vi "fi-constructor.vi"(7 "table.ref in":refnum<vi>, 8 "error in (no error)":errorcluster, 11 "frameInput in":refnum<class "bFrameIO.lvclass">) -> (0 "error out":errorcluster, 3 "frameInput out":refnum<class "bFrameIO.lvclass">)   [LabVIEW 2015, in "bFrameIO.lvclass"]
uses:
  bFrameIO.lvclass
  class.can.table/CAN_table.ctl
  controls/input.params.ctl
  controls/input-states.ctl
  <vilib>/xnet/xnet.llb/XNET Frame CAN.ctl
  <vilib>/xnet/xnet.llb/XNET Frame Type CAN.ctl
  bFrameIO.lvclass/bFrameIO.ctl
  class.can.table/bAPPdata.lvclass
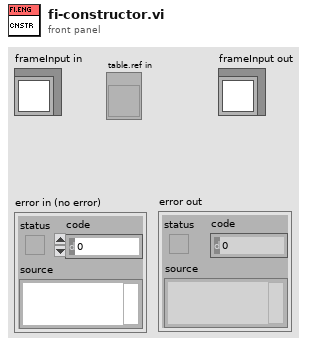
[diagram p1: front panel]
types:
  T1 = typedef "XNET Frame CAN.ctl" = cluster{"timestamp":timestamp, "payload":u8[], "identifier":u32, "type":T2, "extended?":bool, "echo?":bool}
  T2 = typedef "XNET Frame Type CAN.ctl" = u8
  T3 = typedef "bFrameIO.lvclass/input.params.ctl" = cluster{"Interface":refnum<k21>, "CAN_Cluster":refnum<k21>, "input.states":T4, "baudrate":u32}
  T4 = typedef "bFrameIO.lvclass/input-states.ctl" = enum16{"idle", "start", "run", "stop", "exit"}
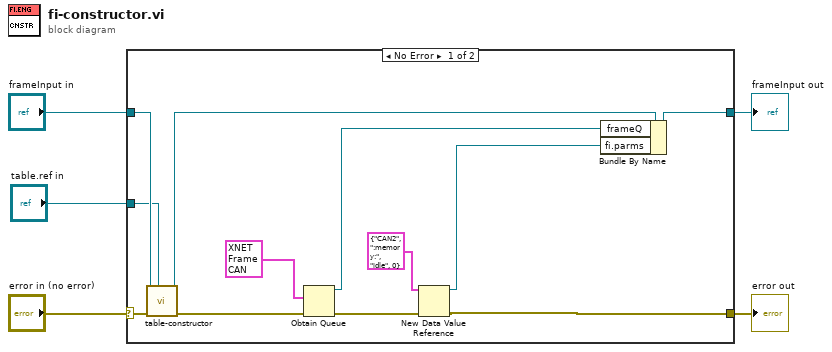
[diagram p0: block diagram]
diagram:
  n1 = case shown="No Error" "error in (no error)" {
    selector: "error in (no error)" -> [w16 w19]
    tunnel: [w11 w19] -> w4
    tunnel: [w17 w18] -> w2
    tunnel: "frameInput in" -> [w9 w18]
    tunnel: "table.ref in" -> [w6 _]
    frame No Error {
      n2 = call "table-constructor.vi"("table.ref in"=w6, "error in (no error)"=w16, "CANtable in"=w9) -> ("error out"=w10:errorcluster, "CANtable out"=w8:refnum<class "bFrameIO.lvclass">)  [unwired: 7 in]
      n3 = Obtain Queue(element data type=T1 {"timestamp"=timestamp(0 s since 1904-01-01), "payload"=[], "identifier"=0, "type"=0, "extended?"=FALSE, "echo?"=FALSE} ("CAN frame"), error in (no error)=w10) -> (queue out=w14:refnum<queue>, error out=w15:errorcluster)  [unwired: 3 in, 1 out]
      n4 = New Data Value Reference(data value=T3 {"Interface"="CAN2", "CAN_Cluster"=":memory:", "input.states"=enum."idle", "baudrate"=0} ("input.parms"), error in=w15) -> (data value reference=w12:refnum<data-value>, error out=w11:errorcluster)
      n5 = Bundle By Name(cluster=w8, "frameQ"=w14, "fi.parms"=w12) -> (w17:refnum<class "bFrameIO.lvclass">)
    }
    frame Error {
    }
  }
  "error out" <- w4
  "frameInput out" <- w2
